vi "Format table.vi"(11 "Table输入":refnum<vi>) -> ()   [LabVIEW 2016, in "斯坦道CODMn.lvlib"]
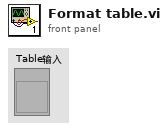
[diagram p1: front panel]
types:
  T1 = cluster{"Font Name:":string, "Size":i16, "Strikeout?":bool, "Italic?":bool, "Underline?":bool, "Outline?":bool, "Shadow?":bool, "Bold?":bool}
  T2 = enum16{"User-specified Font", "Application Font", "System Font", "Dialog Font"}
  T3 = typedef "LVFontTypeDef.ctl" = cluster{"Font Name":string, "Size":u16, "Bold":bool, "Italic":bool, "Underline":bool, "Strikeout":bool, "Color":u32}
  T4 = cluster{"left":i16, "top":i16, "right":i16, "bottom":i16}
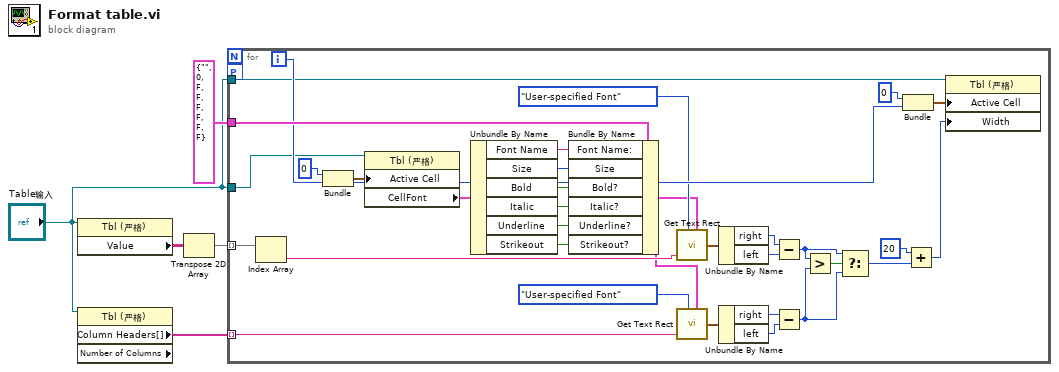
[diagram p0: block diagram]
diagram:
  n1 = property class="Tbl (严格)"(reference="Table输入") -> ("Value"=w5:string[][])  [unwired: 1 in, 2 out]
  n2 = property class="Tbl (严格)" props=["Column Headers[]", "Number of Columns"](reference="Table输入") -> ("Column Headers[]"=w1:string[])  [unwired: 1 in, 3 out]
  n3 = Transpose 2D Array(2D array=w5) -> (transposed array=w4:string[][])
  n4 = for {
    tunnel: w4 -> [w18] mode=indexing
    tunnel: T1 {"Font Name:"="", "Size"=0, "Strikeout?"=FALSE, "Italic?"=FALSE, "Underline?"=FALSE, "Outline?"=FALSE, "Shadow?"=FALSE, "Bold?"=FALSE} ("[user-specified font]") -> [w38]
    tunnel: "Table输入" -> [w32]
    tunnel: "Table输入" -> [w31]
    tunnel: w1 -> [w13] mode=indexing
    workers-P: _ -> [_]
    i -> [w37]
    n5 = Index Array(array=w18) -> (element=w17:string)  [unwired: 1 in]
    n6 = Bundle(0, w37) -> (w19:cluster{i32, i32})  [unwired: 1 in]
    n7 = property on="属性节点" class="Tbl (严格)"(reference=w32, "Active Cell"=w19) -> ("CellFont"=w20:T3)  [unwired: 1 in, 2 out]
    n8 = Unbundle By Name(w20) -> ("Font Name"=w30:string, "Size"=w29:u16, "Bold"=w28:bool, "Italic"=w27:bool, "Underline"=w26:bool, "Strikeout"=w25:bool)
    n9 = Bundle By Name(cluster=w38, "Font Name:"=w30, "Size"=w29, "Bold?"=w28, "Italic?"=w27, "Underline?"=w26, "Strikeout?"=w25) -> (w15:T1)
    n10 = call <vilib>:"Get Text Rect.vi"("desired font(Application)"=T2."User-specified Font", "text"=w17, "[user-specified font]"=w15) -> ("rect"=w23:T4)  [unwired: 6 in]
    n11 = call <vilib>:"Get Text Rect.vi"("desired font(Application)"=T2."User-specified Font", "text"=w13, "[user-specified font]"=w15) -> ("rect"=w10:T4)  [unwired: 6 in]
    n12 = Unbundle By Name(w23) -> ("right"=w22:i16, "left"=w21:i16)
    n13 = Unbundle By Name(w10) -> ("right"=w11:i16, "left"=w12:i16)
    n14 = Subtract(x=w22, y=w21) -> (x-y=w8:i16)
    n15 = Subtract(x=w11, y=w12) -> (x-y=w7:i16)
    n16 = Greater?(x=w8, y=w7) -> (0:w9:bool)
    n17 = Select(t=w8, s=w9, f=w7) -> (s? t:f=w6:i16)
    n18 = Bundle(0, w37) -> (w33:cluster{i32, i32})  [unwired: 1 in]
    n19 = Add(x=i16 20, y=w6) -> (x+y=w34:i16)
    n20 = property on="属性节点" class="Tbl (严格)"(reference=w31, "Active Cell"=w33, "Width"=w34) -> ()  [unwired: 1 in, 2 out]
  }
